vi "closed_loop_arbitrary_analog_stim.vi"() -> ()   [LabVIEW 2014]
uses:
  <vilib>/vision/Measure.llb/Straight Edge Options.ctl
  <vilib>/vision/Measure.llb/Straight Edge Process.ctl
  <vilib>/Platform/TimedLoop/XDataNode/timing_clust.ctl
  <vilib>/Platform/TimedLoop/XDataNode/nitl_modes.ctl
  <vilib>/Platform/TimedLoop/XDataNode/wakeup.ctl
  <vilib>/vision/Measure.llb/Edge Options.ctl
  <vilib>/vision/Measure.llb/Edge Polarity.ctl
  <vilib>/DAQmx/create/channels.llb/DAQmx Create Channel (AO-Voltage-Basic).vi
  <vilib>/DAQmx/write.llb/DAQmx Write (Analog DBL 1Chan 1Samp).vi
  <vilib>/DAQmx/create/channels.llb/DAQmx Create Channel (DO-Digital Output).vi
  <vilib>/DAQmx/write.llb/DAQmx Write (Digital Bool 1Line 1Point).vi
  <vilib>/gmath/statdist.llb/Uniform (Discrete) Random.vi
  <vilib>/Platform/TimedLoop/TimeConversion.llb/rt-rel-time-to-milliseconds.vi
  <vilib>/DAQmx/create/channels.llb/DAQmx Create Channel (DI-Digital Input).vi
  <vilib>/DAQmx/read.llb/DAQmx Read (Digital Bool 1Line 1Point).vi
  <vilib>/platform/TimedLoop/XDataNode/XDataNode.xnode
  <vilib>/vision/driver/NI_Vision_Acquisition_Software.lvlib
  <vilib>/Platform/TimedLoop/XDataNode/XDNodeRunTimeDep.lvlib
  <vilib>/vision/NI_Vision_Development_Module.lvlib
  <vilib>/gmath/NI_Gmath.lvlib
panel:
  out "Slide 5":dbl(slide) scale=0.0..1.0
  out "Stim 4":i32
  in  "Stimulus Folder":path=path "C:/Users/nagellab/Documents/MATLAB/wind_ramps"
  in  "Stimulus Duration (s)":dbl=30.0
  out "Light History":dbl(graph)
  out "Wind History":dbl(graph)
  in  "Initial Orientation (for each trial)":dbl
  out "Light":bool=TRUE
  out "Light Intensity (V)":dbl=3.9 format="%#_13g"
  out "Wind Intensity (V)":dbl=3.1 format="%#_13g"
  out "Wind":bool=TRUE
  out "H0":dbl
  out "Slide 4":dbl(slide) scale=0.0..1.0
  out "Slide 3":dbl(slide) scale=0.0..1.0
  out "Slide 2":dbl(slide) scale=0.0..1.0
  out "Stim 3":i32
  out "Stim 2":i32
  out "Stim 1":i32
  in  "Reversed Tether?":bool=TRUE
  in  "R options":T1={"Number of Lines"=1, "Type"=enum."Best Edge Projection", "Min. Score"=10.0, "Max. Score"=1000.0, "Orientation"=-135.0, "Angle Range"=45.0, "Angle Tolerance"=1.0, "Step Size"=3, "Min. SNR (db)"=0.0, "Min. Points (%)"=25.0, "Hough Iterations"=3} {"Min. Points (%)" min=0.0 max=100.0; "Min. SNR (db)" min=0.0; "Max. Score" min=0.0 max=1024.0; "Min. Score" min=0.0 max=1024.0 step=1.0}
  in  "L options":T1={"Number of Lines"=1, "Type"=enum."Best Edge Projection", "Min. Score"=10.0, "Max. Score"=1000.0, "Orientation"=135.0, "Angle Range"=45.0, "Angle Tolerance"=1.0, "Step Size"=3, "Min. SNR (db)"=0.0, "Min. Points (%)"=25.0, "Hough Iterations"=3} {"Min. Points (%)" min=0.0 max=100.0; "Min. SNR (db)" min=0.0; "Max. Score" min=0.0 max=1024.0; "Min. Score" min=0.0 max=1024.0 step=1.0}
  out "Slide":dbl(slide) scale=0.0..1.0
  out "Motor Error":bool
  in  "Max steps/sample":dbl=6.0
  in  "Step Rate (Hz)":dbl=500.0
  out "Heading (deg)":dbl(graph)
  out "H":dbl format="%.4f"
  out "X (steps/sample)":dbl
  in  "Geneotype":string="w+ Canton-S"
  in  "Starvation Time (hrs)":string="1"
  in  "Age (DSE)":string="4"
  out "Trial End":bool
  in  "Trial Duration (s)":dbl=30.0
  out "Trial":i32 format="%#.3f"
  in  "Number of Trials":i32=20
  in  "Experiment name":string="E1"
  in  "Fly ID":string
  in  "L-R WBA Offset (deg)":dbl format="%#_13g"
  in  "deltaWBA Gain (g, unitless)":dbl=0.04 format="%.4f"
  out "L-R WBA":dbl
  out "deltaWBA":dbl format="%.4f"
  out "Scaled deltaWBA (deg)":dbl(graph)
  out "R WBA":dbl
  out "L WBA":dbl
  out "Image":T3(plugin-control)
  in  "Image Threshold":cluster{"Lower value":sgl, "Upper value":sgl}={"Lower value"=130.0, "Upper value"=255.0} {"Upper value" format="%.2f"; "Lower value" format="%.2f"}
  in  "Data Rate (Hz)":dbl=50.0
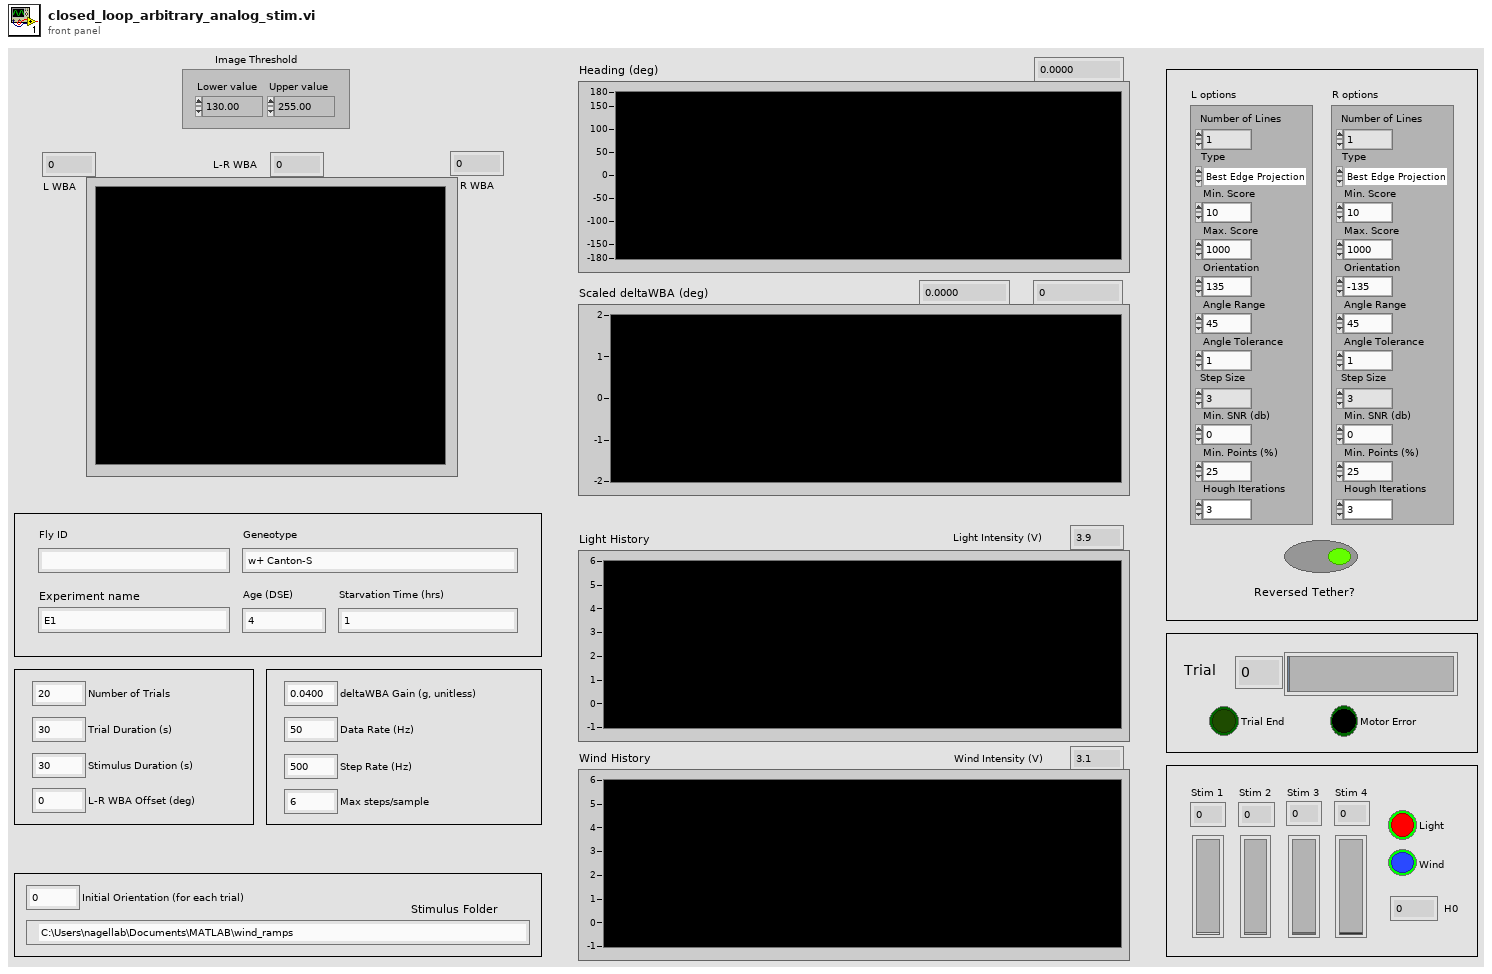
[diagram p1: front panel]
types:
  T1 = typedef "Straight Edge Options.ctl" = cluster{"Number of Lines":i32, "Type":T2, "Min. Score":dbl, "Max. Score":dbl, "Orientation":dbl, "Angle Range":dbl, "Angle Tolerance":dbl, "Step Size":u32, "Min. SNR (db)":dbl, "Min. Points (%)":dbl, "Hough Iterations":i32}
  T2 = typedef "Straight Edge Process.ctl" = enum32{"First Edge Rake", "Best Edge Rake", "Hough Edge Rake", "First Edge Projection", "Best Edge Projection"}
  T3 = typedef "IMAQ Image.ctl" = refnum<image>
  T4 = enum16{"open", "replace", "create", "open or create", "replace or create", "replace or create with confirmation"}
  T5 = typedef "IMAQdx.ctl" = refnum<k21>
  T6 = typedef "IMAQ Rectangle" = cluster{"Left":i32, "Top":i32, "Right":i32, "Bottom":i32, "Rotation":dbl}
  T7 = typedef "ROI Descriptor" = cluster{"Global Rectangle":i32[], "Contours":cluster{"ID":enum32{"External", "Internal"}, "Type":u32, "Coordinates":i32[]}[]}
  T8 = enum16{"big-endian, network order", "native, host order", "little-endian"}
  T9 = typedef "XDNodeRunTimeDep.lvlib/timing_clust.ctl" = cluster{"Expected End [f-1]":u64, "Actual End [f-1]":u64, "Finished Late? [f-1]":bool, "Expected End [i-1]":u64, "Actual End [i-1]":u64, "Finished Late? [i-1]":bool, "Expected Start [i]":u64, "Actual Start [i]":u64, "Expected Start [f]":u64, "Actual Start [f]":u64, "Source Name":string, "Structure Name":string, "Period":i64, "Deadline":i64, "Offset":i64, "Start":i64, "Priority":i32, "Timeout":i32, "Mode":T10, "Wakeup Reason":T11, "Error":errorcluster, "Source Type":string, "Secondary Source Type":string, "Global End Time":u64, "Global Start Time":u64, "Frame Duration":u64, "Iteration Duration":u64, "Assigned CPU":i32, "I/O Scan Engine Mode":u32}
  T10 = typedef "XDNodeRunTimeDep.lvlib/nitl_modes.ctl" = enum32{"No Change", "Process missed periods, maintain original phase", "Discard missed periods, maintain original phase", "Process missed periods, ignore original phase", "Discard missed periods, ignore original phase"}
  T11 = typedef "XDNodeRunTimeDep.lvlib/wakeup.ctl" = enum32{"Normal", "Aborted", "Asynchronous wakeup", "Timing source error", "Timed loop error", "Timeout"}
  T12 = cluster{"y":i32, "y":i32, "y":i32, "y":i32, "y":i32, "y":i32}
  T13 = typedef "Edge Options.ctl" = cluster{"Edge Polarity":T14, "Kernel Size":u32, "Width":u32, "Minimum Edge Strength":sgl, "Interpolation Type":enum32{"Zero Order", "Bilinear", "Quadratic", "Cubic", "Bilinear Fixed"}, "Data Processing Method":enum32{"Average", "Median"}}
  T14 = typedef "Edge Polarity.ctl" = u32
  T15 = cluster{"Search Direction":u32, "Edge Options":T13, "Show Search Area":bool, "Show Search Lines":bool, "Show Edges Found":bool, "Show Result":bool, "Search Area Color":u32, "Search Lines Color":u32, "Edge Locations Color":u32, "Result Color":u32, "Overlay Group Name":string}
  T16 = cluster{"Point1 (Pixels)":cluster{"X":sgl, "Y":sgl}, "Point2 (Pixels)":cluster{"X":sgl, "Y":sgl}, "Point1 (Real-World)":cluster{"X":sgl, "Y":sgl}, "Point2 (Real-World)":cluster{"X":sgl, "Y":sgl}, "Angle (Pixel)":dbl, "Angle (Real-World)":dbl, "Score":dbl, "Straightness":dbl, "Average SNR (db)":dbl, "Calibration Valid":bool}[]
  T17 = cluster{"Straight Edges[0]":cluster{"Point1 (Pixels)":cluster{"X":sgl, "Y":sgl}, "Point2 (Pixels)":cluster{"X":sgl, "Y":sgl}, "Point1 (Real-World)":cluster{"X":sgl, "Y":sgl}, "Point2 (Real-World)":cluster{"X":sgl, "Y":sgl}, "Angle (Pixel)":dbl, "Angle (Real-World)":dbl, "Score":dbl, "Straightness":dbl, "Average SNR (db)":dbl, "Calibration Valid":bool}, "Straight Edges[1]":cluster{"Point1 (Pixels)":cluster{"X":sgl, "Y":sgl}, "Point2 (Pixels)":cluster{"X":sgl, "Y":sgl}, "Point1 (Real-World)":cluster{"X":sgl, "Y":sgl}, "Point2 (Real-World)":cluster{"X":sgl, "Y":sgl}, "Angle (Pixel)":dbl, "Angle (Real-World)":dbl, "Score":dbl, "Straightness":dbl, "Average SNR (db)":dbl, "Calibration Valid":bool}, "Straight Edges[2]":cluster{"Point1 (Pixels)":cluster{"X":sgl, "Y":sgl}, "Point2 (Pixels)":cluster{"X":sgl, "Y":sgl}, "Point1 (Real-World)":cluster{"X":sgl, "Y":sgl}, "Point2 (Real-World)":cluster{"X":sgl, "Y":sgl}, "Angle (Pixel)":dbl, "Angle (Real-World)":dbl, "Score":dbl, "Straightness":dbl, "Average SNR (db)":dbl, "Calibration Valid":bool}, "Straight Edges[3]":cluster{"Point1 (Pixels)":cluster{"X":sgl, "Y":sgl}, "Point2 (Pixels)":cluster{"X":sgl, "Y":sgl}, "Point1 (Real-World)":cluster{"X":sgl, "Y":sgl}, "Point2 (Real-World)":cluster{"X":sgl, "Y":sgl}, "Angle (Pixel)":dbl, "Angle (Real-World)":dbl, "Score":dbl, "Straightness":dbl, "Average SNR (db)":dbl, "Calibration Valid":bool}, "Straight Edges[4]":cluster{"Point1 (Pixels)":cluster{"X":sgl, "Y":sgl}, "Point2 (Pixels)":cluster{"X":sgl, "Y":sgl}, "Point1 (Real-World)":cluster{"X":sgl, "Y":sgl}, "Point2 (Real-World)":cluster{"X":sgl, "Y":sgl}, "Angle (Pixel)":dbl, "Angle (Real-World)":dbl, "Score":dbl, "Straightness":dbl, "Average SNR (db)":dbl, "Calibration Valid":bool}, "Straight Edges[5]":cluster{"Point1 (Pixels)":cluster{"X":sgl, "Y":sgl}, "Point2 (Pixels)":cluster{"X":sgl, "Y":sgl}, "Point1 (Real-World)":cluster{"X":sgl, "Y":sgl}, "Point2 (Real-World)":cluster{"X":sgl, "Y":sgl}, "Angle (Pixel)":dbl, "Angle (Real-World)":dbl, "Score":dbl, "Straightness":dbl, "Average SNR (db)":dbl, "Calibration Valid":bool}, "Straight Edges[6]":cluster{"Point1 (Pixels)":cluster{"X":sgl, "Y":sgl}, "Point2 (Pixels)":cluster{"X":sgl, "Y":sgl}, "Point1 (Real-World)":cluster{"X":sgl, "Y":sgl}, "Point2 (Real-World)":cluster{"X":sgl, "Y":sgl}, "Angle (Pixel)":dbl, "Angle (Real-World)":dbl, "Score":dbl, "Straightness":dbl, "Average SNR (db)":dbl, "Calibration Valid":bool}, "Straight Edges[7]":cluster{"Point1 (Pixels)":cluster{"X":sgl, "Y":sgl}, "Point2 (Pixels)":cluster{"X":sgl, "Y":sgl}, "Point1 (Real-World)":cluster{"X":sgl, "Y":sgl}, "Point2 (Real-World)":cluster{"X":sgl, "Y":sgl}, "Angle (Pixel)":dbl, "Angle (Real-World)":dbl, "Score":dbl, "Straightness":dbl, "Average SNR (db)":dbl, "Calibration Valid":bool}, "Straight Edges[8]":cluster{"Point1 (Pixels)":cluster{"X":sgl, "Y":sgl}, "Point2 (Pixels)":cluster{"X":sgl, "Y":sgl}, "Point1 (Real-World)":cluster{"X":sgl, "Y":sgl}, "Point2 (Real-World)":cluster{"X":sgl, "Y":sgl}, "Angle (Pixel)":dbl, "Angle (Real-World)":dbl, "Score":dbl, "Straightness":dbl, "Average SNR (db)":dbl, "Calibration Valid":bool}}
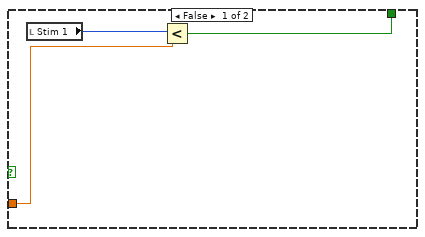
[diagram p2: hidden frame]
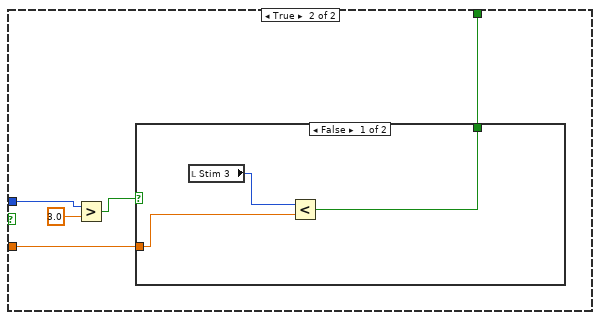
[diagram p3: hidden frame]
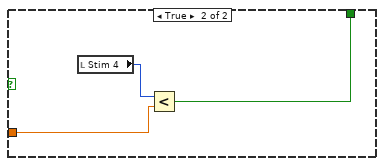
[diagram p4: hidden frame]
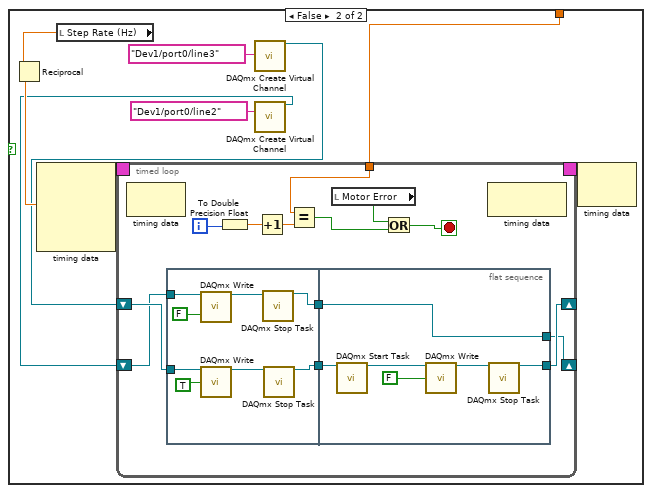
[diagram p6: hidden frame]
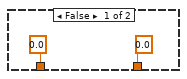
[diagram p7: hidden frame]
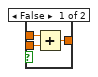
[diagram p8: hidden frame]
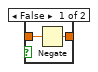
[diagram p9: hidden frame]
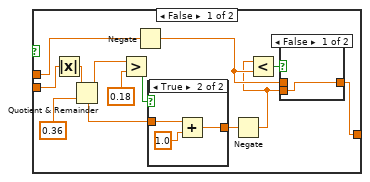
[diagram p10: hidden frame]
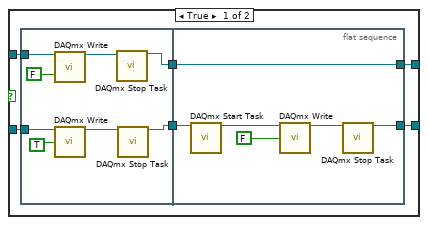
[diagram p16: hidden frame]
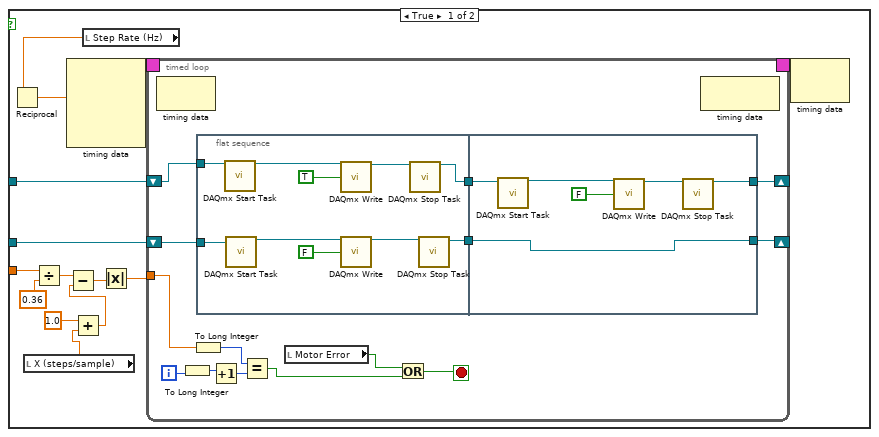
[diagram p18: hidden frame]
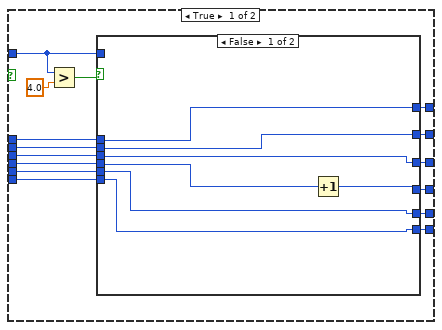
[diagram p19: hidden frame]
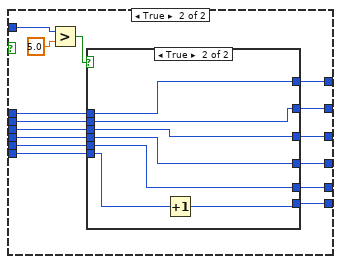
[diagram p20: hidden frame]
diagram:
  w77 = "."
  w79 = "."
  n1 = local read "Wind Intensity (V)"() -> (w24:dbl)
  n2 = local read "Data Rate (Hz)"() -> (w58:dbl)
  n3 = local read "Trial Duration (s)"() -> (w63:dbl)
  n4 = local read "Number of Trials"() -> (w65:i32)
  n5 = local read "Light Intensity (V)"() -> (w22:dbl)
  n6 = local read "deltaWBA Gain (g, unitless)"() -> (w57:dbl)
  n7 = local read "Max steps/sample"() -> (w55:dbl)
  n8 = local read "Step Rate (Hz)"() -> (w56:dbl)
  n9 = local read "Reversed Tether?"() -> (w44:bool)
  n10 = local read "Stimulus Duration (s)"() -> (w13:dbl)
  n11 = Boolean To (0,1)(Boolean=w44) -> (0, 1=w45:i16)
  n12 = To Double Precision Float(number=w45) -> (double precision float=w43:dbl)
  n13 = Number To Fractional String(number=w22, precision (6)=i16 3) -> (F-format string=w20:string)  [unwired: 2 in]
  n14 = Number To Fractional String(number=w65, precision (6)=i16 0) -> (F-format string=w49:string)  [unwired: 2 in]
  n15 = Number To Fractional String(number=w63, precision (6)=i16 0) -> (F-format string=w48:string)  [unwired: 2 in]
  n16 = Number To Fractional String(number=w24, precision (6)=i16 3) -> (F-format string=w21:string)  [unwired: 2 in]
  n17 = Number To Fractional String(number=w58, precision (6)=i16 0) -> (F-format string=w19:string)  [unwired: 2 in]
  n18 = Number To Fractional String(number=w56, precision (6)=i16 0) -> (F-format string=w18:string)  [unwired: 2 in]
  n19 = Number To Fractional String(number=w55, precision (6)=i16 0) -> (F-format string=w17:string)  [unwired: 2 in]
  n20 = Number To Fractional String(number=w57, precision (6)=i16 3) -> (F-format string=w16:string)  [unwired: 2 in]
  n21 = Number To Fractional String(number=w43, precision (6)=i16 0) -> (F-format string=w15:string)  [unwired: 2 in]
  n22 = Number To Fractional String(number=w13, precision (6)=i16 0) -> (F-format string=w12:string)  [unwired: 2 in]
  n23 = Get Date/Time In Seconds() -> (seconds since 1Jan1904=w85:timestamp)
  n24 = Get Date/Time In Seconds() -> (seconds since 1Jan1904=w81:timestamp)
  n25 = Get Date/Time In Seconds() -> (seconds since 1Jan1904=w83:timestamp)
  n26 = call <vilib>:"Space Constant.vi"() -> ("String"=w87:string)
  n27 = Format Date/Time String(time format string (%c)="%d", seconds (now)=w85) -> (date/time string=w76:string)  [unwired: 1 in]
  n28 = Format Date/Time String(time format string (%c)="%m", seconds (now)=w83) -> (date/time string=w78:string)  [unwired: 1 in]
  n29 = Format Date/Time String(time format string (%c)="%Y", seconds (now)=w81) -> (date/time string=w80:string)  [unwired: 1 in]
  n30 = Concatenate Strings(w80, w79, w78, w77, w76) -> (w54:string)
  n31 = Concatenate Strings(w80, w79, w78, w77, w76, w87, "fly_", "Fly ID", "\\") -> (w91:string)
  n32 = String To Path(string=w91) -> (path=w90:path)
  n33 = Build Path(base path=path "E:/TAC DATA ARCHIVE/NewRig/labview/WindRamps", name or relative path=w90) -> (appended path=w95:path)
  n34 = call <vilib>:"IMAQdx Open Camera.vi"("Session In"=refnum<k21> "cam8" ("Camera Name")) -> ("Session Out"=w117:T5)  [unwired: 2 in, 8 out]
  n35 = call <vilib>:"Check if File or Folder Exists.vi"("path"=w95) -> ("file or folder exists?"=w93:bool, "dup path"=w94:path)  [unwired: 8 in, 1 out]
  n36 = call <vilib>:"IMAQdx Configure Grab.vi"("Session In"=w117) -> ("Session Out"=w115:T5)  [unwired: 1 in, 9 out]
  n37 = case shown="False" w93 {
    tunnel: w94 -> [w119 w120]
    tunnel: [w118 w120] -> w99
    frame False {
      n38 = Create Folder(path (use dialog)=w119) -> (created path=w118:path)  [unwired: 2 in, 2 out]
    }
    frame True {
    }
  }
  n39 = call "IMAQ Create"("Image Name"="ROIR") -> ("New Image"=w114:T3)  [unwired: 3 in, 2 out]
  n40 = Concatenate Strings("Experiment name", "\\") -> (w67:string)
  n41 = call <vilib>:"IMAQdx Grab.vi"("Image In"=w114, "Session In"=w115) -> ("Image Out"=w113:T3, "Session Out"=w104:T5)  [unwired: 2 in, 6 out]
  n42 = String To Path(string=w67) -> (path=w96:path)
  n43 = call "IMAQ Select Rectangle"("Prompt"="Select RIGHT ROI for wing angle detection", "Image In"=w113) -> ("Rectangle"=w105:T6)  [unwired: 6 in, 3 out]
  n44 = Build Path(base path=w99, name or relative path=w96) -> (appended path=w100:path)
  n45 = call "IMAQ Convert Rectangle to ROI"("Rectangle"=w105) -> ("ROI Descriptor"=w103:T7)  [unwired: 8 in, 1 out]
  n46 = call <vilib>:"Check if File or Folder Exists.vi"("path"=w100) -> ("file or folder exists?"=w97:bool, "dup path"=w98:path)  [unwired: 8 in, 1 out]
  n47 = call "IMAQ Create"("Image Name"="ROIL") -> ("New Image"=w109:T3)  [unwired: 3 in, 2 out]
  n48 = case shown="False" w97 {
    tunnel: w98 -> [w122 w123]
    tunnel: [w121 w123] -> w5
    frame False {
      n49 = Create Folder(path (use dialog)=w122) -> (created path=w121:path)  [unwired: 2 in, 2 out]
    }
    frame True {
    }
  }
  n50 = call <vilib>:"IMAQdx Grab.vi"("Image In"=w109, "Session In"=w104) -> ("Image Out"=w108:T3, "Session Out"=w102:T5)  [unwired: 2 in, 6 out]
  n51 = String To Path(string="experiment_information") -> (path=w75:path)
  n52 = call "IMAQ Select Rectangle"("Prompt"="Select LEFT ROI for wing angle detection", "Image In"=w108) -> ("Rectangle"=w110:T6)  [unwired: 6 in, 3 out]
  n53 = Build Path(base path=w5, name or relative path=w75) -> (appended path=w72:path)
  n54 = String To Path(string="initial_orientations") -> (path=w34:path)
  n55 = String To Path(string="stimulus_ID") -> (path=w10:path)
  n56 = call "IMAQ Convert Rectangle to ROI"("Rectangle"=w110) -> ("ROI Descriptor"=w101:T7)  [unwired: 8 in, 1 out]
  n57 = Build Path(base path=w5, name or relative path=w34) -> (appended path=w31:path)
  n58 = Build Path(base path=w5, name or relative path=w10) -> (appended path=w7:path)
  n59 = Open/Create/Replace File(file path (use dialog)=w72, operation (0:open)=T4."create", access (0:read/write)=enum16{"read/write", "read-only", "write-only"}."write-only") -> (refnum out=w70:refnum<file>)  [unwired: 3 in, 2 out]
  n60 = Open/Create/Replace File(file path (use dialog)=w31, operation (0:open)=T4."create", access (0:read/write)=enum16{"read/write", "read-only", "write-only"}."write-only") -> (refnum out=w29:refnum<file>)  [unwired: 3 in, 2 out]
  n61 = Open/Create/Replace File(file path (use dialog)=w7, operation (0:open)=T4."create", access (0:read/write)=enum16{"read/write", "read-only", "write-only"}."write-only") -> (refnum out=w3:refnum<file>)  [unwired: 3 in, 2 out]
  n62 = Build Array(w54, "Fly ID", "Experiment name", "Age (DSE)", "Starvation Time (hrs)", w49, w48, w21, w20, w19, w18, w17, w16, w15, w12, "Geneotype") -> (w47:string[])
  n63 = Write to Text File(file (use dialog)=w70, text=w47) -> (refnum out=w69:refnum<file>)  [unwired: 2 in, 2 out]
  n64 = Close File(refnum=w69) -> ()  [unwired: 1 in, 2 out]
  n65 = flat-sequence {
    tunnel: w5 -> [w127]
    tunnel: w101 -> [w128]
    tunnel: w102 -> [w129]
    tunnel: w103 -> [w130]
    tunnel: [w130] -> w42
    tunnel: [w129] -> w40
    tunnel: [w128] -> w38
    tunnel: [w127] -> w36
    tunnel: w29 -> [w125]
    tunnel: [w125] -> w27
    tunnel: [w124] -> w4
    tunnel: w3 -> [w124]
    tunnel: w42 -> [w136]
    tunnel: [w136] -> w41
    tunnel: w40 -> [w135]
    tunnel: [w135] -> w39
    tunnel: w38 -> [w134]
    tunnel: [w134] -> w37
    tunnel: w36 -> [w133]
    tunnel: [w133] -> w35
    tunnel: [w132] -> w28
    tunnel: w27 -> [w132]
    tunnel: w4 -> [w131]
    tunnel: [w131] -> w2
    tunnel: w41 -> [w157]
    tunnel: w39 -> [w156]
    tunnel: w37 -> [w155]
    tunnel: w35 -> [w154]
    tunnel: w28 -> [w148]
    tunnel: [w147] -> w26
    tunnel: w2 -> [w144]
    tunnel: [w143] -> w1
    tunnel: w26 -> [w1087]
    tunnel: w1 -> [w1081]
    frame #0 {
      n66 = One Button Dialog(message="Ensure the stage is at 0 degrees.") -> ()  [unwired: 1 in, 1 out]
    }
    frame #1 {
      n67 = flat-sequence {
        frame #0 {
          n68 = call-poly <vilib>:"DAQmx Create Virtual Channel.vi"("physical channels"=tag "Dev1/ao1") -> ("task out"=w139:refnum<k21>)  [unwired: 13 in, 1 out]
          n69 = call <vilib>:"DAQmx Start Task.vi"("task/channels in"=w139) -> ("task out"=w137:refnum<k21>)  [unwired: 13 in, 1 out]
          n70 = call-poly <vilib>:"DAQmx Write.vi"("task/channels in"=w137, "data"=0.0) -> ("task out"=w138:refnum<k21>)  [unwired: 11 in, 2 out]
          n71 = call <vilib>:"DAQmx Stop Task.vi"("task/channels in"=w138) -> ()  [unwired: 13 in, 2 out]
        }
        frame #1 {
          n72 = Wait (ms)(milliseconds to wait=u32 2000) -> ()  [unwired: 1 out]
        }
      }
    }
    frame #2 {
      n73 = for {
        N: "Number of Trials" -> [_]
        tunnel: w157 -> [w239]
        tunnel: w156 -> [w238]
        tunnel: w155 -> [w237]
        tunnel: w154 -> [w236]
        shift-right: [w215] -> _
        shift-left: 0 ("y") -> [w210]
        shift-right: [w214] -> _
        shift-left: 0 ("y") -> [w208]
        shift-right: [w213] -> _
        shift-left: 0 ("y") -> [w206]
        shift-right: [w212] -> _
        shift-left: 0 ("y") -> [w160]
        shift-right: [w166] -> w147
        shift-left: w148 -> [w184]
        shift-right: [w176] -> _
        shift-left: 0 ("y") -> [w180]
        shift-right: [w177] -> _
        shift-left: 0 ("y") -> [w181]
        shift-right: [w162] -> w143
        shift-left: w144 -> [w165]
        i -> [w233]
        n74 = local read "Number of Trials"() -> (w211:i32)
        n75 = local read "Number of Trials"() -> (w224:i32)
        n76 = Divide(x=w211, y=4) -> (x/y=w158:dbl)
        n77 = Divide(x=w160, y=w158) -> (x/y=→"Slide 5":dbl)
        n78 = Divide(x=w210, y=w158) -> (x/y=→"Slide 2":dbl)
        n79 = Divide(x=w206, y=w158) -> (x/y=→"Slide 4":dbl)
        n80 = Divide(x=w208, y=w158) -> (x/y=→"Slide 3":dbl)
        n81 = flat-sequence {
          tunnel: w223 -> [w268]
          tunnel: w236 -> [w269]
          tunnel: w237 -> [w270]
          tunnel: w238 -> [w271]
          tunnel: w239 -> [w272]
          tunnel: [w272] -> w205
          tunnel: [w271] -> w203
          tunnel: [w270] -> w201
          tunnel: [w269] -> w199
          tunnel: [w268] -> w197
          tunnel: [w260] -> w195
          tunnel: w206 -> [w257]
          tunnel: w160 -> [w256]
          tunnel: w208 -> [w258]
          tunnel: w210 -> [w259]
          tunnel: w158 -> [w255]
          tunnel: [w259] -> w193
          tunnel: [w258] -> w192
          tunnel: [w257] -> w191
          tunnel: [w256] -> w190
          tunnel: w184 -> [w254]
          tunnel: [w254] -> w183
          tunnel: w180 -> [w253]
          tunnel: w181 -> [w252]
          tunnel: [w253] -> w179
          tunnel: [w252] -> w178
          tunnel: w165 -> [w250]
          tunnel: [w250] -> w164
          tunnel: w205 -> [w328]
          tunnel: [w328] -> w204
          tunnel: w203 -> [w327]
          tunnel: [w327] -> w202
          tunnel: w201 -> [w326]
          tunnel: [w326] -> w200
          tunnel: w199 -> [w325]
          tunnel: [w325] -> w198
          tunnel: w197 -> [w324]
          tunnel: [w324] -> w196
          tunnel: w195 -> [w306]
          tunnel: [w323] -> w194
          tunnel: w193 -> [w322]
          tunnel: w192 -> [w321]
          tunnel: w191 -> [w320]
          tunnel: w190 -> [w319]
          tunnel: [w318] -> w189
          tunnel: [w306] -> w188
          tunnel: w183 -> [w317]
          tunnel: [w316] -> w182
          tunnel: w179 -> [w314]
          tunnel: w178 -> [w313]
          tunnel: [w310] -> w174
          tunnel: [w309] -> w173
          tunnel: w164 -> [w308]
          tunnel: [w305] -> w163
          tunnel: [w462] -> w244
          tunnel: [w461] -> w243
          tunnel: [w460] -> w242
          tunnel: [w429] -> w241
          tunnel: w204 -> [w462]
          tunnel: w202 -> [w461]
          tunnel: w200 -> [w460]
          tunnel: w198 -> [w367]
          tunnel: w196 -> [w368]
          tunnel: [w428] -> w232
          tunnel: [w427] -> w229
          tunnel: [w406] -> w228
          tunnel: [w405] -> w227
          tunnel: [w404] -> w221
          tunnel: w194 -> [w403]
          tunnel: [w403] -> w218
          tunnel: w189 -> [w402]
          tunnel: w188 -> [w391]
          tunnel: [w391] -> w187
          tunnel: w182 -> [w364]
          tunnel: w174 -> [w389]
          tunnel: w173 -> [w390]
          tunnel: [w390] -> w172
          tunnel: [w389] -> w171
          tunnel: [w366] -> w170
          tunnel: [w365] -> w169
          tunnel: [w364] -> w166
          tunnel: [w363] -> w162
          tunnel: w163 -> [w363]
          tunnel: w244 -> [w591]
          tunnel: w243 -> [w590]
          tunnel: w242 -> [w589]
          tunnel: w241 -> [w588]
          tunnel: [w587] -> w240
          tunnel: [w586] -> w235
          tunnel: [w585] -> w234
          tunnel: w232 -> [w584]
          tunnel: [w583] -> w231
          tunnel: [w582] -> w230
          tunnel: w229 -> [w581]
          tunnel: w228 -> [w580]
          tunnel: w227 -> [w579]
          tunnel: [w578] -> w226
          tunnel: [w577] -> w225
          tunnel: w221 -> [w570]
          tunnel: [w568] -> w220
          tunnel: [w565] -> w219
          tunnel: w218 -> [w564]
          tunnel: [w564] -> w217
          tunnel: w187 -> [w563]
          tunnel: [w563] -> w186
          tunnel: w172 -> [w561]
          tunnel: w171 -> [w562]
          tunnel: w170 -> [w559]
          tunnel: w169 -> [w558]
          tunnel: [w557] -> w168
          tunnel: [w556] -> w167
          tunnel: w240 -> [w834]
          tunnel: w235 -> [w837]
          tunnel: w234 -> [w836]
          tunnel: w231 -> [w835]
          tunnel: w230 -> [w833]
          tunnel: w226 -> [w832]
          tunnel: w225 -> [w831]
          tunnel: w220 -> [w828]
          tunnel: w219 -> [w826]
          tunnel: w217 -> [w825]
          tunnel: [w825] -> w216
          tunnel: w186 -> [w822]
          tunnel: [w822] -> w185
          tunnel: w168 -> [w821]
          tunnel: w167 -> [w820]
          tunnel: w216 -> [w968]
          tunnel: [w967] -> w215
          tunnel: [w966] -> w214
          tunnel: [w965] -> w213
          tunnel: [w964] -> w212
          tunnel: w185 -> [w958]
          tunnel: [w954] -> w176
          tunnel: [w953] -> w177
          frame #0 {
            n82 = while {
              tunnel: w255 -> [w274]
              tunnel: [w275] -> w260
              stop <- w273 stop-if-true
              n83 = call-poly <vilib>:"Discrete Random.vi"("n"=4, "samples"=1) -> ("uniform (discrete) random data"=w278:i32[])  [unwired: 8 in, 1 out]
              n84 = Index Array(array=w278, index=0) -> (element=w275:i32)
              n85 = Greater?(x=w275, y=2.0) -> (0:w276:bool)
              n86 = case shown="False" w276 {
                tunnel: w275 -> [w282 w296]
                tunnel: w274 -> [w284 w294]
                tunnel: [w283 w293] -> w273
                frame False {
                  n87 = Greater?(x=w282, y=1.0) -> (0:w285:bool)
                  n88 = case shown="True" w285 {
                    tunnel: w284 -> [w288 w291]
                    tunnel: [w287 w290] -> w283
                    frame False {
                      n89 = local read "Stim 1"() -> (w289:i32)
                      n90 = Less?(x=w289, y=w288) -> (x < y?=w287:bool)
                    }
                    frame True {
                      n91 = local read "Stim 2"() -> (w292:i32)
                      n92 = Less?(x=w292, y=w291) -> (x < y?=w290:bool)
                    }
                  }
                }
                frame True {
                  n93 = Greater?(x=w296, y=3.0) -> (0:w295:bool)
                  n94 = case shown="False" w295 {
                    tunnel: w294 -> [w300 w303]
                    tunnel: [w298 w301] -> w293
                    frame False {
                      n95 = local read "Stim 3"() -> (w299:i32)
                      n96 = Less?(x=w299, y=w300) -> (x < y?=w298:bool)
                    }
                    frame True {
                      n97 = local read "Stim 4"() -> (w302:i32)
                      n98 = Less?(x=w302, y=w303) -> (x < y?=w301:bool)
                    }
                  }
                }
              }
            }
            n99 = call-poly <vilib>:"DAQmx Create Virtual Channel.vi"("lines"=tag "Dev1/port0/line0") -> ("task out"=w266:refnum<k21>)  [unwired: 13 in, 1 out]
            n100 = call <vilib>:"DAQmx Start Task.vi"("task/channels in"=w266) -> ("task out"=w265:refnum<k21>)  [unwired: 13 in, 1 out]
            n101 = call-poly <vilib>:"DAQmx Create Virtual Channel.vi"("physical channels"=tag "Dev1/ao1") -> ("task out"=w247:refnum<k21>)  [unwired: 13 in, 1 out]
            n102 = call-poly <vilib>:"DAQmx Write.vi"("task/channels in"=w265, "data"=FALSE) -> ("task out"=w264:refnum<k21>)  [unwired: 11 in, 2 out]
            n103 = call <vilib>:"DAQmx Start Task.vi"("task/channels in"=w247) -> ("task out"=w245:refnum<k21>)  [unwired: 13 in, 1 out]
            n104 = call <vilib>:"DAQmx Stop Task.vi"("task/channels in"=w264) -> ()  [unwired: 13 in, 2 out]
            n105 = call-poly <vilib>:"DAQmx Write.vi"("task/channels in"=w245, "data"=0.0) -> ("task out"=w246:refnum<k21>)  [unwired: 11 in, 2 out]
            n106 = local write "Motor Error"(FALSE ("Trial End")) -> ()
            n107 = call <vilib>:"DAQmx Stop Task.vi"("task/channels in"=w246) -> ()  [unwired: 13 in, 2 out]
            n108 = local write "Trial End"(FALSE ("Trial End")) -> ()
            "H0" <- "Initial Orientation (for each trial)"
          }
          frame #1 {
            n109 = flat-sequence {
              tunnel: [w349] -> w310
              tunnel: [w347] -> w312
              tunnel: w306 -> [w346]
              tunnel: w312 -> [w362]
              frame #0 {
                n110 = Number To Fractional String(number=w346, precision (6)=i16 0) -> (F-format string=w360:string)  [unwired: 2 in]
                n111 = Concatenate Strings("stim" ("string"), w360, "light\\" ("string")) -> (w357:string)
                n112 = Build Path(base path="Stimulus Folder", name or relative path=w357) -> (appended path=w355:path)
                n113 = Open/Create/Replace File(file path (use dialog)=w355, operation (0:open)=T4."open", access (0:read/write)=enum16{"read/write", "read-only", "write-only"}."read-only") -> (refnum out=w352:refnum<file>)  [unwired: 3 in, 2 out]
                n114 = Read from Binary File(5:0.0 ("element"), 9:T8."big-endian, network order" ("byte order (0:big-endian, network order)"), 10:-1 ("count (1)"), 11:w352) -> (2:w349:dbl[], 3:w347:refnum<file>)  [unwired: 2 in, 2 out]
              }
              frame #1 {
                n115 = Close File(refnum=w362) -> ()  [unwired: 1 in, 2 out]
              }
            }
            n116 = flat-sequence {
              tunnel: [w333] -> w309
              tunnel: [w331] -> w311
              tunnel: w306 -> [w330]
              tunnel: w311 -> [w345]
              frame #0 {
                n117 = Number To Fractional String(number=w330, precision (6)=i16 0) -> (F-format string=w343:string)  [unwired: 2 in]
                n118 = local read "Stimulus Folder"() -> (w329:path)
                n119 = Concatenate Strings("stim" ("string"), w343, "wind\\" ("string")) -> (w340:string)
                n120 = Build Path(base path=w329, name or relative path=w340) -> (appended path=w339:path)
                n121 = Open/Create/Replace File(file path (use dialog)=w339, operation (0:open)=T4."open", access (0:read/write)=enum16{"read/write", "read-only", "write-only"}."read-only") -> (refnum out=w336:refnum<file>)  [unwired: 3 in, 2 out]
                n122 = Read from Binary File(5:0.0 ("element"), 9:T8."big-endian, network order" ("byte order (0:big-endian, network order)"), 10:-1 ("count (1)"), 11:w336) -> (2:w333:dbl[], 3:w331:refnum<file>)  [unwired: 2 in, 2 out]
              }
              frame #1 {
                n123 = Close File(refnum=w345) -> ()  [unwired: 1 in, 2 out]
              }
            }
            n124 = local read "H0"() -> (w315:dbl)
            n125 = To Double Precision Float(number=w306) -> (double precision float=w307:dbl)
            n126 = Write to Binary File(file (use dialog)=w308, data=w307) -> (refnum out=w305:refnum<file>)  [unwired: 4 in, 2 out]
            n127 = Write to Binary File(file (use dialog)=w317, data=w315) -> (refnum out=w316:refnum<file>)  [unwired: 4 in, 2 out]
            n128 = call-poly <vilib>:"DAQmx Create Virtual Channel.vi"("lines"=tag "Dev1/port0/line6") -> ("task out"=w318:refnum<k21>)  [unwired: 13 in, 1 out]
            n129 = Bundle("y"=w322, "y"=w321, "y"=w320, "y"=w319, "y"=w314, "y"=w313) -> (w323:T12)  [unwired: 1 in]
          }
          frame #2 {
            n130 = flat-sequence {
              tunnel: w402 -> [w554]
              frame #0 {
              }
              frame #1 {
                n131 = call <vilib>:"DAQmx Start Task.vi"("task/channels in"=w554) -> ("task out"=w553:refnum<k21>)  [unwired: 13 in, 1 out]
                n132 = call-poly <vilib>:"DAQmx Write.vi"("task/channels in"=w553, "data"=TRUE) -> ("task out"=w552:refnum<k21>)  [unwired: 11 in, 2 out]
                n133 = call <vilib>:"DAQmx Stop Task.vi"("task/channels in"=w552) -> ()  [unwired: 13 in, 2 out]
              }
            }
            n134 = local read "H0"() -> (w392:dbl)
            n135 = call <vilib>:"Space Constant.vi"() -> ("String"=w377:string)
            n136 = call <vilib>:"Space Constant.vi"() -> ("String"=w372:string)
            n137 = Number To Fractional String(number=w368, precision (6)=i16 0) -> (F-format string=w378:string)  [unwired: 2 in]
            n138 = Number To Fractional String(number=w368, precision (6)=i16 0) -> (F-format string=w373:string)  [unwired: 2 in]
            n139 = call <vilib>:"Space Constant.vi"() -> ("String"=w432:string)
            n140 = call <vilib>:"Space Constant.vi"() -> ("String"=w452:string)
            n141 = call <vilib>:"Space Constant.vi"() -> ("String"=w419:string)
            n142 = call <vilib>:"Space Constant.vi"() -> ("String"=w443:string)
            n143 = call <vilib>:"Space Constant.vi"() -> ("String"=w409:string)
            n144 = Number To Fractional String(number=w368, precision (6)=i16 0) -> (F-format string=w435:string)  [unwired: 2 in]
            n145 = Number To Fractional String(number=w368, precision (6)=i16 0) -> (F-format string=w455:string)  [unwired: 2 in]
            n146 = Number To Fractional String(number=w368, precision (6)=i16 0) -> (F-format string=w422:string)  [unwired: 2 in]
            n147 = Number To Fractional String(number=w368, precision (6)=i16 0) -> (F-format string=w446:string)  [unwired: 2 in]
            n148 = Number To Fractional String(number=w368, precision (6)=i16 0) -> (F-format string=w412:string)  [unwired: 2 in]
            n149 = Concatenate Strings("trial", w377, w378, w377, "wind_history" ("string")) -> (w369:string)
            n150 = Concatenate Strings("trial", w372, w373, w372, "light_history") -> (w370:string)
            n151 = String To Path(string=w369) -> (path=w388:path)
            n152 = String To Path(string=w370) -> (path=w384:path)
            n153 = Concatenate Strings("trial", w432, w435, w432, "x_data") -> (w437:string)
            n154 = Concatenate Strings("trial", w452, w455, w452, "heading_data") -> (w457:string)
            n155 = Concatenate Strings("trial", w419, w422, w419, "LWBA_data") -> (w424:string)
            n156 = Concatenate Strings("trial", w443, w446, w443, "unfiltered deltaWBA") -> (w448:string)
            n157 = Concatenate Strings("trial", w409, w412, w409, "RWBA_data") -> (w414:string)
            n158 = Build Path(base path=w367, name or relative path=w388) -> (appended path=w385:path)
            n159 = Build Path(base path=w367, name or relative path=w384) -> (appended path=w382:path)
            n160 = String To Path(string=w437) -> (path=w438:path)
            n161 = Divide(x=w392, y=0.36) -> (x/y=w400:dbl)
            n162 = String To Path(string=w457) -> (path=w458:path)
            n163 = String To Path(string=w424) -> (path=w425:path)
            n164 = String To Path(string=w448) -> (path=w449:path)
            n165 = String To Path(string=w414) -> (path=w415:path)
            n166 = To Long Integer(number=w400) -> (32bit integer=w393:i32)
            n167 = Greater Than 0?(x=w393) -> (x > 0?=w399:bool)
            n168 = Not Equal To 0?(x=w393) -> (x != 0?=w394:bool)
            n169 = Build Path(base path=w367, name or relative path=w438) -> (appended path=w431:path)
            n170 = Build Path(base path=w367, name or relative path=w458) -> (appended path=w451:path)
            n171 = Build Path(base path=w367, name or relative path=w425) -> (appended path=w418:path)
            n172 = Build Path(base path=w367, name or relative path=w449) -> (appended path=w442:path)
            n173 = Build Path(base path=w367, name or relative path=w415) -> (appended path=w408:path)
            n174 = To Double Precision Float(number=w393) -> (double precision float=w396:dbl)
            n175 = Absolute Value(x=w393) -> (abs(x)=w398:i32)
            n176 = Multiply(x=0.36, y=w396) -> (x*y=w404:dbl)
            n177 = Open/Create/Replace File(file path (use dialog)=w385, operation (0:open)=T4."create", access (0:read/write)=enum16{"read/write", "read-only", "write-only"}."write-only") -> (refnum out=w366:refnum<file>)  [unwired: 3 in, 2 out]
            n178 = To Double Precision Float(number=w398) -> (double precision float=w397:dbl)
            n179 = case shown="True" w394 {
              tunnel: w399 -> [_ w464]
              tunnel: w397 -> [_ w463]
              frame False {
              }
              frame True {
                n180 = case shown="True" w464 {
                  tunnel: w463 -> [w465 w508]
                  frame True {
                    n181 = local read "Step Rate (Hz)"() -> (w468:dbl)
                    n182 = Reciprocal(x=w468) -> (1/x=w469:dbl)
                    n183 = node-c288(w469) -> (w471:T9)  [unwired: 3 in]
                    n184 = call-poly <vilib>:"DAQmx Create Virtual Channel.vi"("lines"=tag "Dev1/port0/line3") -> ("task out"=w467:refnum<k21>)  [unwired: 13 in, 1 out]
                    n185 = call-poly <vilib>:"DAQmx Create Virtual Channel.vi"("lines"=tag "Dev1/port0/line2") -> ("task out"=w466:refnum<k21>)  [unwired: 13 in, 1 out]
                    n186 = timed-loop {
                      timing: w471 -> [_]
                      timing-out: [_] -> w470
                      shift-right: [w484] -> _
                      shift-left: w467 -> [w482]
                      shift-right: [w483] -> _
                      shift-left: w466 -> [w481]
                      tunnel: w465 -> [w478]
                      i -> [w477]
                      stop <- w476 stop-if-true
                      n187 = node-c288() -> ()  [unwired: 1 in, 1 out]
                      n188 = flat-sequence {
                        tunnel: [w491] -> w486
                        tunnel: [w489] -> w485
                        tunnel: w482 -> [w488]
                        tunnel: w481 -> [w487]
                        tunnel: [w500] -> w484
                        tunnel: [w496] -> w483
                        tunnel: w486 -> [w499]
                        tunnel: w485 -> [w500]
                        frame #0 {
                          n189 = call-poly <vilib>:"DAQmx Write.vi"("task/channels in"=w488, "data"=FALSE) -> ("task out"=w490:refnum<k21>)  [unwired: 11 in, 2 out]
                          n190 = call-poly <vilib>:"DAQmx Write.vi"("task/channels in"=w487, "data"=TRUE) -> ("task out"=w492:refnum<k21>)  [unwired: 11 in, 2 out]
                          n191 = call <vilib>:"DAQmx Stop Task.vi"("task/channels in"=w490) -> ("task out"=w489:refnum<k21>)  [unwired: 13 in, 1 out]
                          n192 = call <vilib>:"DAQmx Stop Task.vi"("task/channels in"=w492) -> ("task out"=w491:refnum<k21>)  [unwired: 13 in, 1 out]
                        }
                        frame #1 {
                          n193 = call <vilib>:"DAQmx Start Task.vi"("task/channels in"=w499) -> ("task out"=w498:refnum<k21>)  [unwired: 13 in, 1 out]
                          n194 = call-poly <vilib>:"DAQmx Write.vi"("task/channels in"=w498, "data"=FALSE) -> ("task out"=w497:refnum<k21>)  [unwired: 11 in, 2 out]
                          n195 = call <vilib>:"DAQmx Stop Task.vi"("task/channels in"=w497) -> ("task out"=w496:refnum<k21>)  [unwired: 13 in, 1 out]
                        }
                      }
                      n196 = To Double Precision Float(number=w477) -> (double precision float=w479:dbl)
                      n197 = Increment(x=w479) -> (x+1=w480:dbl)
                      n198 = local read "Motor Error"() -> (w474:bool)
                      n199 = Equal?(x=w478, y=w480) -> (x = y?=w475:bool)
                      n200 = Or(x=w474, y=w475) -> (x .or. y?=w476:bool)
                      n201 = node-c288() -> ()  [unwired: 1 in, 1 out]
                    }
                    n202 = node-c288(w470) -> ()  [unwired: 1 out]
                  }
                  frame False {
                    n203 = local read "Step Rate (Hz)"() -> (w511:dbl)
                    n204 = Reciprocal(x=w511) -> (1/x=w512:dbl)
                    n205 = node-c288(w512) -> (w514:T9)  [unwired: 3 in]
                    n206 = call-poly <vilib>:"DAQmx Create Virtual Channel.vi"("lines"=tag "Dev1/port0/line3") -> ("task out"=w510:refnum<k21>)  [unwired: 13 in, 1 out]
                    n207 = call-poly <vilib>:"DAQmx Create Virtual Channel.vi"("lines"=tag "Dev1/port0/line2") -> ("task out"=w509:refnum<k21>)  [unwired: 13 in, 1 out]
                    n208 = timed-loop {
                      timing: w514 -> [_]
                      timing-out: [_] -> w513
                      shift-right: [w526] -> _
                      shift-left: w510 -> [w527]
                      shift-right: [w524] -> _
                      shift-left: w509 -> [w525]
                      tunnel: w508 -> [w520]
                      i -> [w519]
                      stop <- w518 stop-if-true
                      n209 = node-c288() -> ()  [unwired: 1 in, 1 out]
                      n210 = flat-sequence {
                        tunnel: [w534] -> w529
                        tunnel: [w532] -> w528
                        tunnel: w525 -> [w531]
                        tunnel: w527 -> [w530]
                        tunnel: [w543] -> w524
                        tunnel: [w539] -> w526
                        tunnel: w529 -> [w542]
                        tunnel: w528 -> [w543]
                        frame #0 {
                          n211 = call-poly <vilib>:"DAQmx Write.vi"("task/channels in"=w531, "data"=FALSE) -> ("task out"=w533:refnum<k21>)  [unwired: 11 in, 2 out]
                          n212 = call-poly <vilib>:"DAQmx Write.vi"("task/channels in"=w530, "data"=TRUE) -> ("task out"=w535:refnum<k21>)  [unwired: 11 in, 2 out]
                          n213 = call <vilib>:"DAQmx Stop Task.vi"("task/channels in"=w533) -> ("task out"=w532:refnum<k21>)  [unwired: 13 in, 1 out]
                          n214 = call <vilib>:"DAQmx Stop Task.vi"("task/channels in"=w535) -> ("task out"=w534:refnum<k21>)  [unwired: 13 in, 1 out]
                        }
                        frame #1 {
                          n215 = call <vilib>:"DAQmx Start Task.vi"("task/channels in"=w542) -> ("task out"=w541:refnum<k21>)  [unwired: 13 in, 1 out]
                          n216 = call-poly <vilib>:"DAQmx Write.vi"("task/channels in"=w541, "data"=FALSE) -> ("task out"=w540:refnum<k21>)  [unwired: 11 in, 2 out]
                          n217 = call <vilib>:"DAQmx Stop Task.vi"("task/channels in"=w540) -> ("task out"=w539:refnum<k21>)  [unwired: 13 in, 1 out]
                        }
                      }
                      n218 = To Double Precision Float(number=w519) -> (double precision float=w522:dbl)
                      n219 = Increment(x=w522) -> (x+1=w523:dbl)
                      n220 = Equal?(x=w520, y=w523) -> (x = y?=w521:bool)
                      n221 = local read "Motor Error"() -> (w517:bool)
                      n222 = Or(x=w517, y=w521) -> (x .or. y?=w518:bool)
                      n223 = node-c288() -> ()  [unwired: 1 in, 1 out]
                    }
                    n224 = node-c288(w513) -> ()  [unwired: 1 out]
                  }
                }
              }
            }
            n225 = Open/Create/Replace File(file path (use dialog)=w382, operation (0:open)=T4."create", access (0:read/write)=enum16{"read/write", "read-only", "write-only"}."write-only") -> (refnum out=w365:refnum<file>)  [unwired: 3 in, 2 out]
            n226 = Open/Create/Replace File(file path (use dialog)=w431, operation (0:open)=T4."create", access (0:read/write)=enum16{"read/write", "read-only", "write-only"}."write-only") -> (refnum out=w429:refnum<file>)  [unwired: 3 in, 2 out]
            n227 = Open/Create/Replace File(file path (use dialog)=w451, operation (0:open)=T4."create", access (0:read/write)=enum16{"read/write", "read-only", "write-only"}."write-only") -> (refnum out=w428:refnum<file>)  [unwired: 3 in, 2 out]
            n228 = Open/Create/Replace File(file path (use dialog)=w418, operation (0:open)=T4."create", access (0:read/write)=enum16{"read/write", "read-only", "write-only"}."write-only") -> (refnum out=w406:refnum<file>)  [unwired: 3 in, 2 out]
            n229 = Open/Create/Replace File(file path (use dialog)=w442, operation (0:open)=T4."create", access (0:read/write)=enum16{"read/write", "read-only", "write-only"}."write-only") -> (refnum out=w427:refnum<file>)  [unwired: 3 in, 2 out]
            n230 = Open/Create/Replace File(file path (use dialog)=w408, operation (0:open)=T4."create", access (0:read/write)=enum16{"read/write", "read-only", "write-only"}."write-only") -> (refnum out=w405:refnum<file>)  [unwired: 3 in, 2 out]
            n231 = local write "Heading (deg)"(w404) -> ()
            n232 = local write "H"(w404) -> ()
          }
          frame #3 {
            n233 = call-poly <vilib>:"DAQmx Create Virtual Channel.vi"("lines"=tag "Dev1/port0/line3") -> ("task out"=w575:refnum<k21>)  [unwired: 13 in, 1 out]
            n234 = call-poly <vilib>:"DAQmx Create Virtual Channel.vi"("lines"=tag "Dev1/port0/line2") -> ("task out"=w576:refnum<k21>)  [unwired: 13 in, 1 out]
            n235 = call-poly <vilib>:"DAQmx Create Virtual Channel.vi"("physical channels"=tag "Dev1/ao1") -> ("task out"=w569:refnum<k21>)  [unwired: 13 in, 1 out]
            n236 = call-poly <vilib>:"DAQmx Create Virtual Channel.vi"("physical channels"=tag "Dev1/ao0") -> ("task out"=w566:refnum<k21>)  [unwired: 13 in, 1 out]
            n237 = Reciprocal(x="Data Rate (Hz)") -> (1/x=w560:dbl)
            n238 = call-poly <vilib>:"DAQmx Create Virtual Channel.vi"("lines"=tag "Dev1/port0/line1") -> ("task out"=w571:refnum<k21>)  [unwired: 13 in, 1 out]
            n239 = node-c288(w560) -> (w594:T9)  [unwired: 3 in]
            n240 = timed-loop {
              timing: w594 -> [_]
              timing-out: [_] -> w593
              tunnel: w591 -> [w687]
              tunnel: w590 -> [w688]
              tunnel: w589 -> [w686]
              shift-right: [w670] -> w585
              shift-left: w576 -> [w672]
              shift-right: [w671] -> w586
              shift-left: w575 -> [w673]
              tunnel: w588 -> [w685]
              tunnel: [w684] -> w587
              shift-right: [w682] -> _
              shift-left: w570 -> [w683]
              tunnel: w584 -> [w681]
              tunnel: [w680] -> w583
              tunnel: [w679] -> w582
              tunnel: w581 -> [w678]
              tunnel: w580 -> [w677]
              tunnel: w579 -> [w676]
              tunnel: [w675] -> w578
              tunnel: [w674] -> w577
              shift-right: [w666] -> _
              shift-left: w571 -> [w669]
              shift-right: [w610] -> _
              shift-left: _ -> [w624]
              shift-right: [w619] -> w568
              shift-left: w569 -> [w622]
              shift-right: [w611] -> w565
              shift-left: w566 -> [w612]
              tunnel: w562 -> [w609]
              tunnel: w561 -> [w608]
              tunnel: w559 -> [w603]
              tunnel: w558 -> [w602]
              tunnel: [w601] -> w557
              tunnel: [w600] -> w556
              i -> [w604]
              stop <- w663 stop-if-true
              w652 = T15 {"Search Direction"=0, "Edge Options"={"Edge Polarity"=0, "Kernel Size"=3, "Width"=3, "Minimum Edge Strength"=2.0, "Interpolation Type"=enum."Bilinear Fixed", "Data Processing Method"=enum."Average"}, "Show Search Area"=TRUE, "Show Search Lines"=TRUE, "Show Edges Found"=TRUE, "Show Result"=TRUE, "Search Area Color"=65280, "Search Lines Color"=255, "Edge Locations Color"=16776960, "Result Color"=16711680, "Overlay Group Name"=""} ("Options")
              n241 = node-c288() -> ()  [unwired: 1 in, 1 out]
              n242 = To Double Precision Float(number=w604) -> (double precision float=w628:dbl)
              n243 = local read "Data Rate (Hz)"() -> (w599:dbl)
              n244 = local read "Data Rate (Hz)"() -> (w643:dbl)
              n245 = Increment(x=w628) -> (x+1=w639:dbl)
              n246 = call <vilib>:"DAQmx Start Task.vi"("task/channels in"=w622) -> ("task out"=w621:refnum<k21>)  [unwired: 13 in, 1 out]
              n247 = Multiply(x=w599, y="Stimulus Duration (s)") -> (x*y=w605:dbl)
              n248 = Less?(x=w604, y=w605) -> (x < y?=w607:bool)
              n249 = case shown="True" w607 {
                tunnel: w609 -> [_ w695]
                tunnel: w608 -> [_ w694]
                tunnel: w604 -> [_ w693]
                tunnel: [0.0 ("element") w692] -> w596
                tunnel: [0.0 ("element") w691] -> w595
                frame False {
                }
                frame True {
                  n250 = Index Array(array=w695, index=w693) -> (element=w692:dbl)
                  n251 = Index Array(array=w694, index=w693) -> (element=w691:dbl)
                }
              }
              "Wind History" <- w595
              "Light History" <- w596
              "Wind Intensity (V)" <- w595
              "Light Intensity (V)" <- w596
              n252 = call <vilib>:"DAQmx Start Task.vi"("task/channels in"=w669) -> ("task out"=w668:refnum<k21>)  [unwired: 13 in, 1 out]
              n253 = Divide(x=w639, y=w643) -> (x/y=w642:dbl)
              n254 = call-poly <vilib>:"DAQmx Write.vi"("task/channels in"=w621, "data"=w595) -> ("task out"=w620:refnum<k21>)  [unwired: 11 in, 2 out]
              n255 = call "IMAQ Create"("Image Name"="flyim") -> ("New Image"=w662:T3)  [unwired: 3 in, 2 out]
              n256 = Greater?(x=w642, y="Trial Duration (s)") -> (0:→"Trial End":bool)
              n257 = call <vilib>:"DAQmx Stop Task.vi"("task/channels in"=w620) -> ("task out"=w619:refnum<k21>)  [unwired: 13 in, 1 out]
              n258 = call-poly <vilib>:"DAQmx Read.vi"("task/channels in"=w668) -> ("task out"=w667:refnum<k21>, "data"=→"Motor Error":bool)  [unwired: 12 in, 1 out]
              n259 = call <vilib>:"IMAQdx Grab.vi"("Wait for Next Buffer? (Yes)"=FALSE, "Image In"=w662, "Session In"=w688) -> ("Image Out"=w653:T3)  [unwired: 1 in, 7 out]
              n260 = call "IMAQ Threshold"("Keep/Replace Value (Replace)"=FALSE, "Range"="Image Threshold", "Image Src"=w653) -> ("Image Dst Out"=w658:T3)  [unwired: 7 in, 1 out]
              n261 = call <vilib>:"DAQmx Stop Task.vi"("task/channels in"=w667) -> ("task out"=w666:refnum<k21>)  [unwired: 13 in, 1 out]
              n262 = call "IMAQ Find Edge"("Line Fit Options"="L options", "Options"=w652, "ROI Descriptor"=w687, "Image"=w658) -> ("Straight Edges"=w655:T16, "Image Out"=w657:T3)  [unwired: 4 in, 2 out]
              n263 = Write to Binary File(file (use dialog)=w603, data=w595) -> (refnum out=w601:refnum<file>)  [unwired: 4 in, 2 out]
              n264 = Write to Binary File(file (use dialog)=w602, data=w596) -> (refnum out=w600:refnum<file>)  [unwired: 4 in, 2 out]
              n265 = call <vilib>:"DAQmx Start Task.vi"("task/channels in"=w612) -> ("task out"=w598:refnum<k21>)  [unwired: 13 in, 1 out]
              n266 = call "IMAQ Find Edge"("Line Fit Options"="R options", "Options"=w652, "ROI Descriptor"=w686, "Image"=w657) -> ("Straight Edges"=w654:T16, "Image Out"=→"Image":T3)  [unwired: 4 in, 2 out]
              n267 = Array To Cluster(array=w654) -> (cluster=w645:T17)
              n268 = Array To Cluster(array=w655) -> (cluster=w644:T17)
              n269 = call-poly <vilib>:"DAQmx Write.vi"("task/channels in"=w598, "data"=w596) -> ("task out"=w597:refnum<k21>)  [unwired: 11 in, 2 out]
              n270 = Unbundle By Name(w645) -> ("Straight Edges[0].Angle (Pixel)"=w650:dbl)
              n271 = Unbundle By Name(w644) -> ("Straight Edges[0].Angle (Pixel)"=w651:dbl)
              n272 = call <vilib>:"DAQmx Stop Task.vi"("task/channels in"=w597) -> ("task out"=w611:refnum<k21>)  [unwired: 13 in, 1 out]
              n273 = Absolute Value(x=w650) -> (abs(x)=w629:dbl)
              "L WBA" <- w629
              n274 = Absolute Value(x=w651) -> (abs(x)=w630:dbl)
              "R WBA" <- w630
              n275 = Write to Binary File(file (use dialog)=w676, data=w630) -> (refnum out=w675:refnum<file>)  [unwired: 4 in, 2 out]
              n276 = Write to Binary File(file (use dialog)=w677, data=w629) -> (refnum out=w674:refnum<file>)  [unwired: 4 in, 2 out]
              n277 = Subtract(x=w629, y=w630) -> (x-y=w648:dbl)
              "L-R WBA" <- w648
              n278 = case shown="True" "Reversed Tether?" {
                tunnel: w648 -> [w698 w700]
                tunnel: [w697 w699] -> w647
                tunnel: "L-R WBA Offset (deg)" -> [w696 w701]
                frame False {
                  n279 = Add ("Add.vi")(x=w698, y=w696) -> (x+y=w697:dbl)
                }
                frame True {
                  n280 = Subtract(x=w700, y=w701) -> (x-y=w699:dbl)
                }
              }
              n281 = Multiply(x=w647, y="deltaWBA Gain (g, unitless)") -> (x*y=w649:dbl)
              n282 = case shown="True" "Reversed Tether?" {
                tunnel: w649 -> [w703 w704]
                tunnel: [w702 w704] -> w616
                frame False {
                  n283 = Negate(x=w703) -> (-x=w702:dbl)
                }
                frame True {
                }
              }
              "Scaled deltaWBA (deg)" <- w616
              "deltaWBA" <- w616
              n284 = Greater Or Equal To 0?(x=w616) -> (x >= 0?=w617:bool)
              n285 = case shown="True" w617 {
                tunnel: [w715 w732] -> w610
                tunnel: "Max steps/sample" -> [w714 w728]
                tunnel: w616 -> [w708 w727]
                frame False {
                  n286 = Absolute Value(x=w708) -> (abs(x)=w709:dbl)
                  n287 = Quotient & Remainder(x=w709, y=0.36) -> (x-y*floor(x/y)=w707:dbl, floor(x/y)=w710:dbl)
                  n288 = Greater?(x=w707, y=0.18) -> (0:w711:bool)
                  n289 = Negate(x=w714) -> (-x=w716:dbl)
                  n290 = case shown="True" w711 {
                    tunnel: w710 -> [w718 w721]
                    tunnel: [w718 w719] -> w706
                    frame False {
                    }
                    frame True {
                      n291 = Add(x=w721, y=1.0) -> (x+y=w719:dbl)
                    }
                  }
                  n292 = Negate(x=w706) -> (-x=w705:dbl)
                  n293 = Less?(x=w705, y=w716) -> (x < y?=w717:bool)
                  n294 = case shown="False" w717 {
                    tunnel: w716 -> [_ w723]
                    tunnel: [w722 w723] -> w715
                    tunnel: w705 -> [w722 _]
                    frame False {
                    }
                    frame True {
                    }
                  }
                }
                frame True {
                  n295 = Quotient & Remainder(x=w727, y=0.36) -> (x-y*floor(x/y)=w725:dbl, floor(x/y)=w730:dbl)
                  n296 = Greater?(x=w725, y=0.18) -> (0:w726:bool)
                  n297 = case shown="True" w726 {
                    tunnel: w730 -> [w734 w737]
                    tunnel: [w734 w735] -> w731
                    frame False {
                    }
                    frame True {
                      n298 = Add(x=w737, y=1.0) -> (x+y=w735:dbl)
                    }
                  }
                  n299 = Greater?(x=w731, y=w728) -> (0:w733:bool)
                  n300 = case shown="False" w733 {
                    tunnel: w728 -> [_ w739]
                    tunnel: [w738 w739] -> w732
                    tunnel: w731 -> [w738 _]
                    frame False {
                    }
                    frame True {
                    }
                  }
                }
              }
              "X (steps/sample)" <- w610
              n301 = Multiply(x=0.36 ("y"), y=w610) -> (x*y=w631:dbl)
              n302 = Add ("Add.vi")(x=w631, y=w683) -> (x+y=w635:dbl)
              n303 = Add(x=w635, y=180.0 ("x")) -> (x+y=w636:dbl)
              n304 = Quotient & Remainder(x=w636, y=360.0) -> (x-y*floor(x/y)=w637:dbl)  [unwired: 1 out]
              n305 = Subtract(x=w637, y=180.0) -> (x-y=w682:dbl)
              "H" <- w682
              "Heading (deg)" <- w682
              n306 = Write to Binary File(file (use dialog)=w681, data=w682) -> (refnum out=w680:refnum<file>)  [unwired: 4 in, 2 out]
              n307 = Write to Binary File(file (use dialog)=w678, data=w616) -> (refnum out=w684:refnum<file>)  [unwired: 4 in, 2 out]
              n308 = Write to Binary File(file (use dialog)=w685, data=w610) -> (refnum out=w679:refnum<file>)  [unwired: 4 in, 2 out]
              n309 = Not Equal To 0?(x=w624) -> (x != 0?=w625:bool)
              n310 = case shown="True" w625 {
                tunnel: w673 -> [w741 w748]
                tunnel: w672 -> [w740 w747]
                tunnel: w624 -> [_ w746]
                tunnel: [w740 w745] -> w670
                tunnel: [w741 w744] -> w671
                frame False {
                }
                frame True {
                  n311 = Reciprocal(x="Step Rate (Hz)") -> (1/x=w742:dbl)
                  n312 = node-c288(w742) -> (w750:T9)  [unwired: 3 in]
                  n313 = timed-loop {
                    timing: w750 -> [_]
                    timing-out: [_] -> w749
                    tunnel: w746 -> [w764]
                    shift-right: [w757] -> w744
                    shift-left: w748 -> [w761]
                    shift-right: [w756] -> w745
                    shift-left: w747 -> [w759]
                    i -> [w755]
                    stop <- w753 stop-if-true
                    n314 = node-c288() -> ()  [unwired: 1 in, 1 out]
                    n315 = To Double Precision Float(number=w755) -> (double precision float=w754:dbl)
                    n316 = Absolute Value(x=w764) -> (abs(x)=w763:dbl)
                    n317 = call <vilib>:"DAQmx Start Task.vi"("task/channels in"=w761) -> ("task out"=w760:refnum<k21>)  [unwired: 13 in, 1 out]
                    n318 = call <vilib>:"DAQmx Start Task.vi"("task/channels in"=w759) -> ("task out"=w758:refnum<k21>)  [unwired: 13 in, 1 out]
                    n319 = Increment(x=w754) -> (x+1=w762:dbl)
                    n320 = Greater Than 0?(x=w764) -> (x > 0?=w765:bool)
                    n321 = Equal?(x=w763, y=w762) -> (x = y?=w752:bool)
                    n322 = case shown="False" w765 {
                      tunnel: [w768 w788] -> w757
                      tunnel: [w769 w789] -> w756
                      tunnel: w758 -> [w771 w791]
                      tunnel: w760 -> [w770 w790]
                      frame True {
                        n323 = flat-sequence {
                          tunnel: w771 -> [w779]
                          tunnel: w770 -> [w778]
                          tunnel: [w774] -> w767
                          tunnel: [w772] -> w766
                          tunnel: [w785] -> w768
                          tunnel: [w781] -> w769
                          tunnel: w767 -> [w784]
                          tunnel: w766 -> [w785]
                          frame #0 {
                            n324 = call-poly <vilib>:"DAQmx Write.vi"("task/channels in"=w778, "data"=FALSE) -> ("task out"=w773:refnum<k21>)  [unwired: 11 in, 2 out]
                            n325 = call-poly <vilib>:"DAQmx Write.vi"("task/channels in"=w779, "data"=TRUE) -> ("task out"=w775:refnum<k21>)  [unwired: 11 in, 2 out]
                            n326 = call <vilib>:"DAQmx Stop Task.vi"("task/channels in"=w773) -> ("task out"=w772:refnum<k21>)  [unwired: 13 in, 1 out]
                            n327 = call <vilib>:"DAQmx Stop Task.vi"("task/channels in"=w775) -> ("task out"=w774:refnum<k21>)  [unwired: 13 in, 1 out]
                          }
                          frame #1 {
                            n328 = call <vilib>:"DAQmx Start Task.vi"("task/channels in"=w784) -> ("task out"=w783:refnum<k21>)  [unwired: 13 in, 1 out]
                            n329 = call-poly <vilib>:"DAQmx Write.vi"("task/channels in"=w783, "data"=FALSE) -> ("task out"=w782:refnum<k21>)  [unwired: 11 in, 2 out]
                            n330 = call <vilib>:"DAQmx Stop Task.vi"("task/channels in"=w782) -> ("task out"=w781:refnum<k21>)  [unwired: 13 in, 1 out]
                          }
                        }
                      }
                      frame False {
                        n331 = flat-sequence {
                          tunnel: w791 -> [w799]
                          tunnel: w790 -> [w798]
                          tunnel: [w794] -> w787
                          tunnel: [w792] -> w786
                          tunnel: [w801] -> w788
                          tunnel: [w800] -> w789
                          tunnel: w787 -> [w800]
                          tunnel: w786 -> [w802]
                          frame #0 {
                            n332 = call-poly <vilib>:"DAQmx Write.vi"("task/channels in"=w798, "data"=TRUE) -> ("task out"=w793:refnum<k21>)  [unwired: 11 in, 2 out]
                            n333 = call-poly <vilib>:"DAQmx Write.vi"("task/channels in"=w799, "data"=FALSE) -> ("task out"=w795:refnum<k21>)  [unwired: 11 in, 2 out]
                            n334 = call <vilib>:"DAQmx Stop Task.vi"("task/channels in"=w793) -> ("task out"=w792:refnum<k21>)  [unwired: 13 in, 1 out]
                            n335 = call <vilib>:"DAQmx Stop Task.vi"("task/channels in"=w795) -> ("task out"=w794:refnum<k21>)  [unwired: 13 in, 1 out]
                          }
                          frame #1 {
                            n336 = call <vilib>:"DAQmx Start Task.vi"("task/channels in"=w802) -> ("task out"=w805:refnum<k21>)  [unwired: 13 in, 1 out]
                            n337 = call-poly <vilib>:"DAQmx Write.vi"("task/channels in"=w805, "data"=FALSE) -> ("task out"=w804:refnum<k21>)  [unwired: 11 in, 2 out]
                            n338 = call <vilib>:"DAQmx Stop Task.vi"("task/channels in"=w804) -> ("task out"=w801:refnum<k21>)  [unwired: 13 in, 1 out]
                          }
                        }
                      }
                    }
                    n339 = local read "Motor Error"() -> (w751:bool)
                    n340 = Or(x=w752, y=w751) -> (x .or. y?=w753:bool)
                    n341 = node-c288() -> ()  [unwired: 1 in, 1 out]
                  }
                  n342 = node-c288(w749) -> ()  [unwired: 1 out]
                }
              }
              n343 = local read "Motor Error"() -> (w664:bool)
              n344 = local read "Trial End"() -> (w665:bool)
              n345 = Or(x=w665, y=w664) -> (x .or. y?=w663:bool)
              n346 = node-c288() -> ()  [unwired: 1 in, 1 out]
            }
            n347 = node-c288(w593) -> ()  [unwired: 1 out]
          }
          frame #4 {
            n348 = local read "H"() -> (w827:dbl)
            n349 = Close File(refnum=w821) -> ()  [unwired: 1 in, 2 out]
            n350 = Close File(refnum=w820) -> ()  [unwired: 1 in, 2 out]
            n351 = Absolute Value(x=w827) -> (abs(x)=w824:dbl)
            n352 = Close File(refnum=w834) -> ()  [unwired: 1 in, 2 out]
            n353 = Close File(refnum=w833) -> ()  [unwired: 1 in, 2 out]
            n354 = Close File(refnum=w832) -> ()  [unwired: 1 in, 2 out]
            n355 = Close File(refnum=w831) -> ()  [unwired: 1 in, 2 out]
            n356 = Close File(refnum=w835) -> ()  [unwired: 1 in, 2 out]
            n357 = Greater Than 0?(x=w827) -> (x > 0?=w830:bool)
            n358 = To Long Integer(number=w824) -> (32bit integer=w823:i32)
            n359 = Not Equal To 0?(x=w823) -> (x != 0?=w829:bool)
            n360 = case shown="True" w829 {
              tunnel: w837 -> [_ w850]
              tunnel: w836 -> [_ w849]
              tunnel: w830 -> [_ w848]
              tunnel: w827 -> [_ w847]
              frame False {
              }
              frame True {
                n361 = case shown="False" w848 {
                  tunnel: w850 -> [w861 w912]
                  tunnel: w849 -> [w860 w911]
                  tunnel: w847 -> [w858 w909]
                  frame True {
                    n362 = local read "X (steps/sample)"() -> (w852:dbl)
                    n363 = Divide(x=w858, y=0.36) -> (x/y=w854:dbl)
                    n364 = Add(x=1.0, y=w852) -> (x+y=w853:dbl)
                    n365 = Subtract(x=w854, y=w853) -> (x-y=w856:dbl)
                    n366 = local read "Step Rate (Hz)"() -> (w859:dbl)
                    n367 = Reciprocal(x=w859) -> (1/x=w862:dbl)
                    n368 = node-c288(w862) -> (w864:T9)  [unwired: 3 in]
                    n369 = Absolute Value(x=w856) -> (abs(x)=w855:dbl)
                    n370 = timed-loop {
                      timing: w864 -> [_]
                      timing-out: [_] -> w863
                      shift-right: [w876] -> _
                      shift-left: w860 -> [w874]
                      shift-right: [w877] -> _
                      shift-left: w861 -> [w875]
                      tunnel: w855 -> [w868]
                      i -> [w866]
                      stop <- w871 stop-if-true
                      n371 = node-c288() -> ()  [unwired: 1 in, 1 out]
                      n372 = To Long Integer(number=w866) -> (32bit integer=w865:i32)
                      n373 = To Long Integer(number=w868) -> (32bit integer=w867:i32)
                      n374 = flat-sequence {
                        tunnel: w875 -> [w884]
                        tunnel: w874 -> [w882]
                        tunnel: [w887] -> w873
                        tunnel: [w885] -> w872
                        tunnel: [w894] -> w876
                        tunnel: [w889] -> w877
                        tunnel: w873 -> [w892]
                        tunnel: w872 -> [w894]
                        frame #0 {
                          n375 = call <vilib>:"DAQmx Start Task.vi"("task/channels in"=w884) -> ("task out"=w883:refnum<k21>)  [unwired: 13 in, 1 out]
                          n376 = call <vilib>:"DAQmx Start Task.vi"("task/channels in"=w882) -> ("task out"=w881:refnum<k21>)  [unwired: 13 in, 1 out]
                          n377 = call-poly <vilib>:"DAQmx Write.vi"("task/channels in"=w883, "data"=TRUE) -> ("task out"=w888:refnum<k21>)  [unwired: 11 in, 2 out]
                          n378 = call-poly <vilib>:"DAQmx Write.vi"("task/channels in"=w881, "data"=FALSE) -> ("task out"=w886:refnum<k21>)  [unwired: 11 in, 2 out]
                          n379 = call <vilib>:"DAQmx Stop Task.vi"("task/channels in"=w888) -> ("task out"=w887:refnum<k21>)  [unwired: 13 in, 1 out]
                          n380 = call <vilib>:"DAQmx Stop Task.vi"("task/channels in"=w886) -> ("task out"=w885:refnum<k21>)  [unwired: 13 in, 1 out]
                        }
                        frame #1 {
                          n381 = call <vilib>:"DAQmx Start Task.vi"("task/channels in"=w892) -> ("task out"=w891:refnum<k21>)  [unwired: 13 in, 1 out]
                          n382 = call-poly <vilib>:"DAQmx Write.vi"("task/channels in"=w891, "data"=FALSE) -> ("task out"=w890:refnum<k21>)  [unwired: 11 in, 2 out]
                          n383 = call <vilib>:"DAQmx Stop Task.vi"("task/channels in"=w890) -> ("task out"=w889:refnum<k21>)  [unwired: 13 in, 1 out]
                        }
                      }
                      n384 = Increment(x=w865) -> (x+1=w878:i32)
                      n385 = Equal?(x=w867, y=w878) -> (x = y?=w869:bool)
                      n386 = local read "Motor Error"() -> (w870:bool)
                      n387 = Or(x=w870, y=w869) -> (x .or. y?=w871:bool)
                      n388 = node-c288() -> ()  [unwired: 1 in, 1 out]
                    }
                    n389 = node-c288(w863) -> ()  [unwired: 1 out]
                  }
                  frame False {
                    n390 = local read "X (steps/sample)"() -> (w904:dbl)
                    n391 = Divide(x=w909, y=0.36) -> (x/y=w907:dbl)
                    n392 = Add(x=1.0, y=w904) -> (x+y=w902:dbl)
                    n393 = local read "Step Rate (Hz)"() -> (w910:dbl)
                    n394 = Reciprocal(x=w910) -> (1/x=w913:dbl)
                    n395 = node-c288(w913) -> (w915:T9)  [unwired: 3 in]
                    n396 = Subtract(x=w907, y=w902) -> (x-y=w906:dbl)
                    n397 = Absolute Value(x=w906) -> (abs(x)=w905:dbl)
                    n398 = timed-loop {
                      timing: w915 -> [_]
                      timing-out: [_] -> w914
                      shift-right: [w927] -> _
                      shift-left: w911 -> [w925]
                      shift-right: [w928] -> _
                      shift-left: w912 -> [w926]
                      tunnel: w905 -> [w917]
                      i -> [w919]
                      stop <- w922 stop-if-true
                      n399 = node-c288() -> ()  [unwired: 1 in, 1 out]
                      n400 = To Long Integer(number=w917) -> (32bit integer=w916:i32)
                      n401 = To Long Integer(number=w919) -> (32bit integer=w918:i32)
                      n402 = flat-sequence {
                        tunnel: w926 -> [w935]
                        tunnel: w925 -> [w933]
                        tunnel: [w938] -> w924
                        tunnel: [w936] -> w923
                        tunnel: [w941] -> w927
                        tunnel: [w940] -> w928
                        tunnel: w924 -> [w940]
                        tunnel: w923 -> [w942]
                        frame #0 {
                          n403 = call <vilib>:"DAQmx Start Task.vi"("task/channels in"=w935) -> ("task out"=w934:refnum<k21>)  [unwired: 13 in, 1 out]
                          n404 = call <vilib>:"DAQmx Start Task.vi"("task/channels in"=w933) -> ("task out"=w932:refnum<k21>)  [unwired: 13 in, 1 out]
                          n405 = call-poly <vilib>:"DAQmx Write.vi"("task/channels in"=w934, "data"=FALSE) -> ("task out"=w939:refnum<k21>)  [unwired: 11 in, 2 out]
                          n406 = call-poly <vilib>:"DAQmx Write.vi"("task/channels in"=w932, "data"=TRUE) -> ("task out"=w937:refnum<k21>)  [unwired: 11 in, 2 out]
                          n407 = call <vilib>:"DAQmx Stop Task.vi"("task/channels in"=w939) -> ("task out"=w938:refnum<k21>)  [unwired: 13 in, 1 out]
                          n408 = call <vilib>:"DAQmx Stop Task.vi"("task/channels in"=w937) -> ("task out"=w936:refnum<k21>)  [unwired: 13 in, 1 out]
                        }
                        frame #1 {
                          n409 = call <vilib>:"DAQmx Start Task.vi"("task/channels in"=w942) -> ("task out"=w944:refnum<k21>)  [unwired: 13 in, 1 out]
                          n410 = call-poly <vilib>:"DAQmx Write.vi"("task/channels in"=w944, "data"=FALSE) -> ("task out"=w943:refnum<k21>)  [unwired: 11 in, 2 out]
                          n411 = call <vilib>:"DAQmx Stop Task.vi"("task/channels in"=w943) -> ("task out"=w941:refnum<k21>)  [unwired: 13 in, 1 out]
                        }
                      }
                      n412 = Increment(x=w918) -> (x+1=w929:i32)
                      n413 = Equal?(x=w916, y=w929) -> (x = y?=w921:bool)
                      n414 = local read "Motor Error"() -> (w920:bool)
                      n415 = Or(x=w920, y=w921) -> (x .or. y?=w922:bool)
                      n416 = node-c288() -> ()  [unwired: 1 in, 1 out]
                    }
                    n417 = node-c288(w914) -> ()  [unwired: 1 out]
                  }
                }
              }
            }
            n418 = flat-sequence {
              tunnel: w828 -> [w845]
              tunnel: w826 -> [w840]
              frame #0 {
                n419 = call <vilib>:"DAQmx Start Task.vi"("task/channels in"=w840) -> ("task out"=w842:refnum<k21>)  [unwired: 13 in, 1 out]
                n420 = call <vilib>:"DAQmx Start Task.vi"("task/channels in"=w845) -> ("task out"=w844:refnum<k21>)  [unwired: 13 in, 1 out]
                n421 = call-poly <vilib>:"DAQmx Write.vi"("task/channels in"=w842, "data"=0.0) -> ("task out"=w841:refnum<k21>)  [unwired: 11 in, 2 out]
                n422 = call-poly <vilib>:"DAQmx Write.vi"("task/channels in"=w844, "data"=0.0) -> ("task out"=w843:refnum<k21>)  [unwired: 11 in, 2 out]
                n423 = call <vilib>:"DAQmx Stop Task.vi"("task/channels in"=w841) -> ()  [unwired: 13 in, 2 out]
                n424 = call <vilib>:"DAQmx Stop Task.vi"("task/channels in"=w843) -> ()  [unwired: 13 in, 2 out]
              }
              frame #1 {
                n425 = Wait (ms)(milliseconds to wait=u32 2000) -> ()  [unwired: 1 out]
              }
            }
          }
          frame #5 {
            n426 = Unbundle(w968) -> ("y"=w962:i32, "y"=w961:i32, "y"=w960:i32, "y"=w959:i32, "y"=w956:i32, "y"=w955:i32)
            n427 = Greater?(x=w958, y=3.0) -> (0:w957:bool)
            n428 = case shown="False" w957 {
              tunnel: [w988 w1039] -> w967
              tunnel: [w987 w1038] -> w966
              tunnel: [w986 w1037] -> w965
              tunnel: [w985 w1036] -> w964
              tunnel: w962 -> [w984 w1035]
              tunnel: w961 -> [w983 w1034]
              tunnel: w960 -> [w982 w1033]
              tunnel: w959 -> [w981 w1032]
              tunnel: w958 -> [w974 w1025]
              tunnel: w956 -> [w978 w1029]
              tunnel: w955 -> [w977 w1028]
              tunnel: [w976 w1027] -> w954
              tunnel: [w975 w1026] -> w953
              frame True {
                n429 = Greater?(x=w974, y=4.0) -> (0:w979:bool)
                n430 = case shown="False" w979 {
                  tunnel: w984 -> [w989 w1008]
                  tunnel: w983 -> [w990 w1007]
                  tunnel: w982 -> [w991 w1006]
                  tunnel: w981 -> [w994 w1005]
                  tunnel: [w989 w1001] -> w988
                  tunnel: [w990 w1002] -> w987
                  tunnel: [w991 w1004] -> w986
                  tunnel: [w995 w1003] -> w985
                  tunnel: w974 -> [_ w1000]
                  tunnel: w978 -> [w992 w999]
                  tunnel: w977 -> [w993 w998]
                  tunnel: [w992 w997] -> w976
                  tunnel: [w993 w996] -> w975
                  frame False {
                    n431 = Increment(x=w994) -> (x+1=w995:i32)
                  }
                  frame True {
                    n432 = Greater?(x=w1000, y=5.0) -> (0:w1009:bool)
                    n433 = case shown="True" w1009 {
                      tunnel: w1008 -> [w1017 w1024]
                      tunnel: w1007 -> [w1016 w1023]
                      tunnel: w1006 -> [w1014 w1022]
                      tunnel: w1005 -> [w1015 w1020]
                      tunnel: [w1017 w1024] -> w1001
                      tunnel: [w1016 w1023] -> w1002
                      tunnel: [w1014 w1022] -> w1004
                      tunnel: [w1015 w1020] -> w1003
                      tunnel: w999 -> [w1013 w1021]
                      tunnel: w998 -> [w1011 w1019]
                      tunnel: [w1012 w1021] -> w997
                      tunnel: [w1011 w1018] -> w996
                      frame False {
                        n434 = Increment(x=w1013) -> (x+1=w1012:i32)
                      }
                      frame True {
                        n435 = Increment(x=w1019) -> (x+1=w1018:i32)
                      }
                    }
                  }
                }
              }
              frame False {
                n436 = Greater?(x=w1025, y=1.0) -> (0:w1030:bool)
                n437 = case shown="True" w1030 {
                  tunnel: w1035 -> [w1041 w1059]
                  tunnel: w1034 -> [w1043 w1058]
                  tunnel: w1033 -> [w1044 w1057]
                  tunnel: w1032 -> [w1042 w1056]
                  tunnel: [w1040 w1052] -> w1039
                  tunnel: [w1043 w1053] -> w1038
                  tunnel: [w1044 w1055] -> w1037
                  tunnel: [w1042 w1054] -> w1036
                  tunnel: w1025 -> [_ w1051]
                  tunnel: w1029 -> [w1045 w1050]
                  tunnel: w1028 -> [w1046 w1049]
                  tunnel: [w1045 w1048] -> w1027
                  tunnel: [w1046 w1047] -> w1026
                  frame False {
                    n438 = Increment(x=w1041) -> (x+1=w1040:i32)
                  }
                  frame True {
                    n439 = Greater?(x=w1051, y=2.0) -> (0:w1060:bool)
                    n440 = case shown="True" w1060 {
                      tunnel: w1059 -> [w1068 w1075]
                      tunnel: w1058 -> [w1063 w1074]
                      tunnel: w1057 -> [w1066 w1069]
                      tunnel: w1056 -> [w1067 w1072]
                      tunnel: [w1068 w1075] -> w1052
                      tunnel: [w1062 w1074] -> w1053
                      tunnel: [w1066 w1070] -> w1055
                      tunnel: [w1067 w1072] -> w1054
                      tunnel: w1050 -> [w1064 w1073]
                      tunnel: w1049 -> [w1065 w1071]
                      tunnel: [w1064 w1073] -> w1048
                      tunnel: [w1065 w1071] -> w1047
                      frame False {
                        n441 = Increment(x=w1063) -> (x+1=w1062:i32)
                      }
                      frame True {
                        n442 = Increment(x=w1069) -> (x+1=w1070:i32)
                      }
                    }
                  }
                }
              }
            }
            n443 = call-poly <vilib>:"DAQmx Create Virtual Channel.vi"("lines"=tag "Dev1/port0/line0") -> ("task out"=w972:refnum<k21>)  [unwired: 13 in, 1 out]
            n444 = call <vilib>:"DAQmx Start Task.vi"("task/channels in"=w972) -> ("task out"=w971:refnum<k21>)  [unwired: 13 in, 1 out]
            n445 = call-poly <vilib>:"DAQmx Write.vi"("task/channels in"=w971, "data"=TRUE) -> ("task out"=w970:refnum<k21>)  [unwired: 11 in, 2 out]
            n446 = call <vilib>:"DAQmx Stop Task.vi"("task/channels in"=w970) -> ()  [unwired: 13 in, 2 out]
          }
        }
        n447 = Increment(x=w233) -> (x+1=w223:i32)
        "Trial" <- w223
        n448 = Divide(x=w223, y=w224) -> (x/y=→"Slide":dbl)
        "Stim 1" <- w210
        "Stim 2" <- w208
        "Stim 3" <- w206
        "Stim 4" <- w160
      }
    }
    frame #3 {
      n449 = Close File(refnum=w1087) -> ()  [unwired: 1 in, 2 out]
      n450 = Close File(refnum=w1081) -> ()  [unwired: 1 in, 2 out]
      n451 = call-poly <vilib>:"DAQmx Create Virtual Channel.vi"("physical channels"=tag "Dev1/ao1") -> ("task out"=w1090:refnum<k21>)  [unwired: 13 in, 1 out]
      n452 = call-poly <vilib>:"DAQmx Create Virtual Channel.vi"("physical channels"=tag "Dev1/ao0") -> ("task out"=w1084:refnum<k21>)  [unwired: 13 in, 1 out]
      n453 = call-poly <vilib>:"DAQmx Create Virtual Channel.vi"("lines"=tag "Dev1/port0/line6") -> ("task out"=w1078:refnum<k21>)  [unwired: 13 in, 1 out]
      n454 = call <vilib>:"DAQmx Start Task.vi"("task/channels in"=w1090) -> ("task out"=w1092:refnum<k21>)  [unwired: 13 in, 1 out]
      n455 = call <vilib>:"DAQmx Start Task.vi"("task/channels in"=w1084) -> ("task out"=w1086:refnum<k21>)  [unwired: 13 in, 1 out]
      n456 = call <vilib>:"DAQmx Start Task.vi"("task/channels in"=w1078) -> ("task out"=w1080:refnum<k21>)  [unwired: 13 in, 1 out]
      n457 = call-poly <vilib>:"DAQmx Write.vi"("task/channels in"=w1092, "data"=5.0) -> ("task out"=w1091:refnum<k21>)  [unwired: 11 in, 2 out]
      n458 = call-poly <vilib>:"DAQmx Write.vi"("task/channels in"=w1086, "data"=5.0) -> ("task out"=w1085:refnum<k21>)  [unwired: 11 in, 2 out]
      n459 = call-poly <vilib>:"DAQmx Write.vi"("task/channels in"=w1080, "data"=FALSE) -> ("task out"=w1079:refnum<k21>)  [unwired: 11 in, 2 out]
      n460 = call <vilib>:"DAQmx Stop Task.vi"("task/channels in"=w1091) -> ()  [unwired: 13 in, 2 out]
      n461 = call <vilib>:"DAQmx Stop Task.vi"("task/channels in"=w1085) -> ()  [unwired: 13 in, 2 out]
      n462 = call <vilib>:"DAQmx Stop Task.vi"("task/channels in"=w1079) -> ()  [unwired: 13 in, 2 out]
    }
  }
